vi "Create Events.vi"(8 "error in (no error)":errorcluster, 11 "SMO":refnum<class "SMO.lvclass">) -> (0 "error out":errorcluster, 3 "SMO out":refnum<class "SMO.lvclass">)   [LabVIEW 2021, in "smo.lvlib" / "SMO.lvclass"]
uses:
  SMO.lvclass
  SMO.lvclass/SMO.ctl
panel:
  # "For instructions on how to use the JKI State Machine Objects, examples and video tutorials, visit:\nhttp://jki.net/state-machine-objects/\n\nJKI State Machine Objects™\nhttp://jki.net/state-machine-objects/\nCopyright (C) 2005-2015, JKI <info@jki.net>\nALL RIGHTS RESERVED"
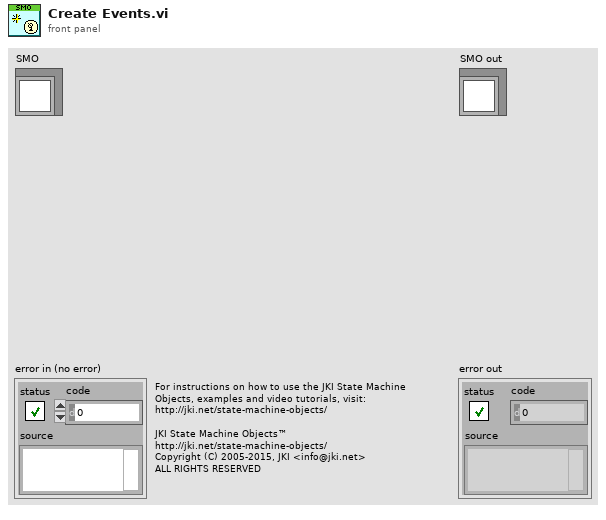
[diagram p1: front panel]
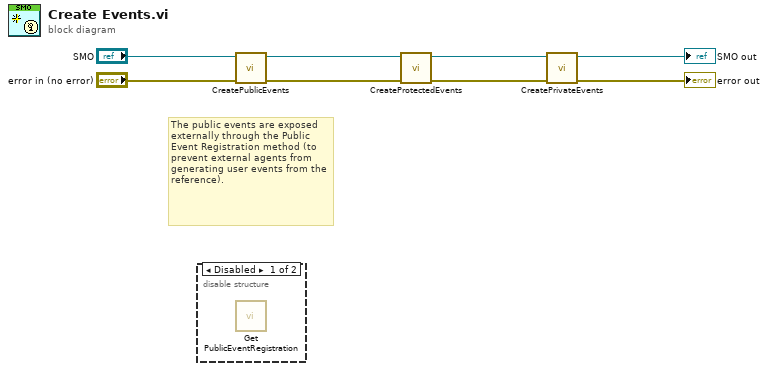
[diagram p0: block diagram]
diagram:
  # "The public events are exposed externally through the Public Event Registration method (to prevent external agents from generating user events from the reference)."
  n1 = disable-structure shown="Disabled" {
    frame Disabled {
      n2 = call "Get PublicEventRegistration.vi"() -> ()  [unwired: 9 in, 3 out]
    }
    frame Enabled {
    }
  }
  n3 = call-dynamic "CreatePublicEvents.vi"("error in (no error)"="error in (no error)", "SMO"="SMO") -> ("error out"=w5:errorcluster, "SMO out"=w6:refnum<class "SMO.lvclass">)  [unwired: 8 in]
  n4 = call-dynamic "CreateProtectedEvents.vi"("error in (no error)"=w5, "SMO"=w6) -> ("error out"=w2:errorcluster, "SMO out"=w4:refnum<class "SMO.lvclass">)  [unwired: 8 in]
  n5 = call-dynamic "CreatePrivateEvents.vi"("error in (no error)"=w2, "SMO"=w4) -> ("error out"=→"error out":errorcluster, "SMO out"=→"SMO out":refnum<class "SMO.lvclass">)  [unwired: 8 in]
